vi "Set Inline Buffer.vi"(8 "error in (no error)":errorcluster, 10 "Command Parameters":T1, 11 "Dispatcher in":refnum<class "Dispatcher Thread.lvclass">) -> (0 "error out":errorcluster, 3 "Dispatcher out":refnum<class "Dispatcher Thread.lvclass">)   [LabVIEW 2017, in "DSF Core.lvlib" / "Dispatcher Thread.lvclass"]
uses:
  Dispatcher Thread.lvclass
  Interfaces/Dispatcher/Parameters.ctl
  Interfaces/Dispatcher/Response Data.ctl
  Interfaces/Dispatcher/Response.ctl
  Dispatcher Thread.lvclass/Dispatcher Thread.ctl
  Thread Pool/Plugin Interface Pool.lvclass/Plugin Interface Pool.ctl
  Interfaces/Dispatcher/Write.vi
  Interfaces/Dispatcher/Write Dispatcher Response.vi
  Interfaces/Plugin/Plugin Interface.lvclass
  Thread Pool/Plugin Interface Pool.lvclass
  Interfaces/Dispatcher/Dispatcher Interface.lvclass
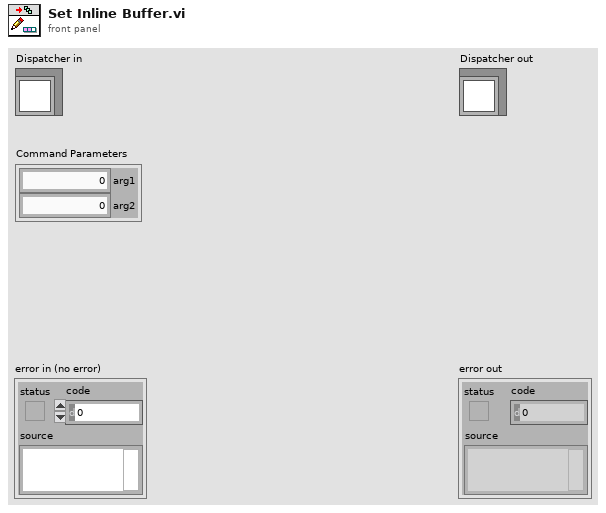
[diagram p1: front panel]
types:
  T1 = typedef "DSF Core.lvlib/Dispatcher Interface.lvclass/Parameters.ctl" = cluster{"arg1":u64, "arg2":u64}
  T2 = typedef "DSF Core.lvlib/Dispatcher Interface.lvclass/Response.ctl" = enum8{"General Ack", "Error", "Shutting Down"}
  T3 = typedef "DSF Core.lvlib/Dispatcher Interface.lvclass/Response Data.ctl" = cluster{"Response":T2, "Parameters":T1}
  T4 = typedef "DSF Core.lvlib/Dispatcher Thread.lvclass/Plugin Settings.ctl" = cluster{"Transfer Group threads":i32[], "Plugin Thread Pool":refnum<class "Plugin Interface Pool.lvclass">}
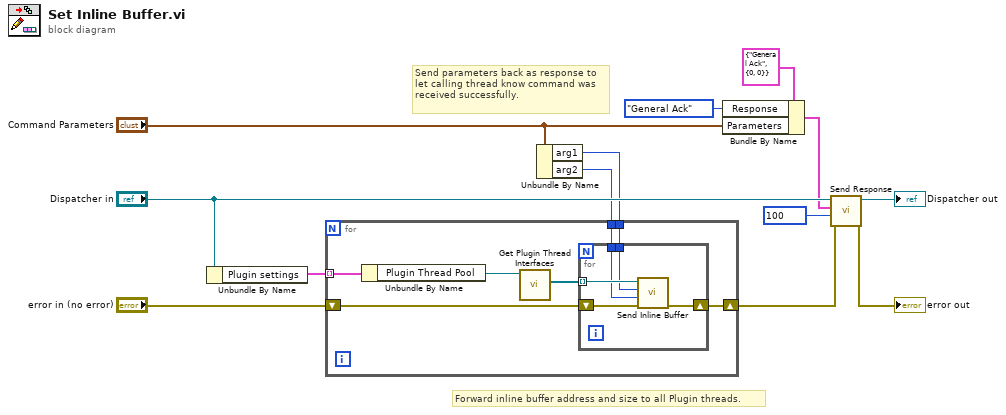
[diagram p0: block diagram]
diagram:
  # "Send parameters back as response to let calling thread know command was received successfully."
  # "Forward inline buffer address and size to all Plugin threads."
  n1 = Unbundle By Name("Dispatcher in") -> ("Plugin settings"=w13:T4[])
  n2 = Unbundle By Name("Command Parameters") -> ("arg1"=w3:u64, "arg2"=w2:u64)
  n3 = for {
    tunnel: w13 -> [w15] mode=indexing
    shift-right: [w19] -> w6
    shift-left: "error in (no error)" -> [w18]
    tunnel: w2 -> [w17]
    tunnel: w3 -> [w16]
    n4 = Unbundle By Name(w15) -> ("Plugin Thread Pool"=w14:refnum<class "Plugin Interface Pool.lvclass">)
    n5 = call "Get Plugin Thread Interfaces.vi"("Plugin Interface Pool in"=w14) -> ("Plugin Thread Interfaces"=w20:refnum<class "Plugin Interface.lvclass">[])  [unwired: 9 in, 1 out]
    n6 = for {
      tunnel: w20 -> [w25] mode=indexing
      shift-right: [w24] -> w19
      shift-left: w18 -> [w23]
      tunnel: w17 -> [w21]
      tunnel: w16 -> [w22]
      n7 = call "Send Inline Buffer.vi"("error in (no error)"=w23, "size"=w21, "address"=w22, "Plugin Interface in"=w25) -> ("error out"=w24:errorcluster)  [unwired: 6 in, 1 out]
    }
  }
  n8 = Bundle By Name(cluster=T3 {"Response"=enum."General Ack", "Parameters"={"arg1"=0, "arg2"=0}} ("response"), "Response"=Response."General Ack", "Parameters"="Command Parameters") -> (w7:T3)
  n9 = call "Send Response.vi"("error in (no error)"=w6, "timeout in ms (0)"=100, "response"=w7, "Dispatcher in"="Dispatcher in") -> ("error out"=→"error out":errorcluster, "Dispatcher out"=→"Dispatcher out":refnum<class "Dispatcher Thread.lvclass">)  [unwired: 6 in]
